vi "Execute Step.vi"(6 "Message Queue":refnum<queue>, 8 "error in (no error)":errorcluster, 9 "Step":T1, 11 "Status":T2) -> (0 "error out":errorcluster, 3 "Status":T2)   [LabVIEW 2012]
doc: "This VI will:\n- confirm that the vehicle is in the correct position\n- update the proper indicators on the console\n- set the vehicle in position light to green\n- indicate the time remaining to the console (continuously update as the step is executing)\n- once the step is complete, the appropriate indicators will be updated (for the steps)\n-- if the vehicle needs to move before more steps can be executed (or at the end of a cycle) exit and set waiting status to vehicle position"
uses:
  Architecture/Message Queue/Message Cluster.ctl
  Architecture/Message Queue/Message Queue.lvlib
  Simulated Console/Controls/Button state.ctl
  Controls/Controller Status.ctl
  Controls/Steps.ctl
  Controls/Stations.ctl
  Controls/Waiting States.ctl
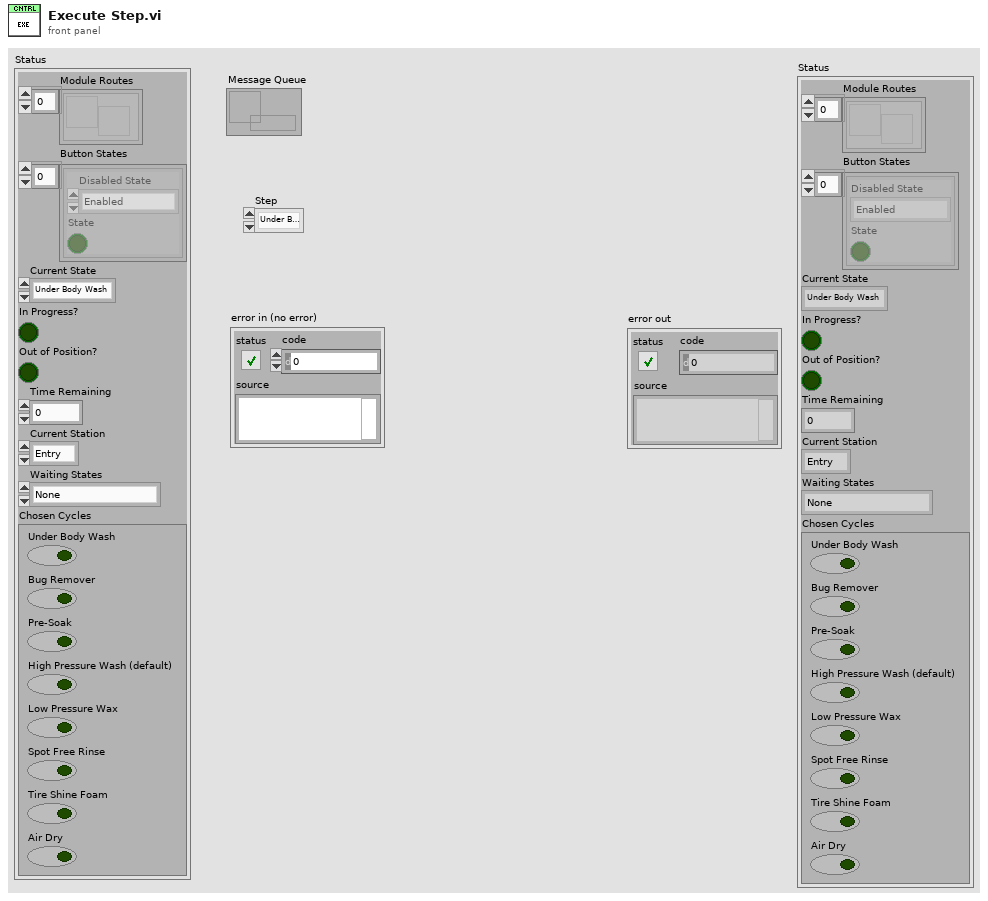
[diagram p1: front panel]
types:
  T1 = typedef "Steps.ctl" = enum16{"Under Body Wash", "Bug Remover", "Pre-Soak", "High Pressure Wash", "Low Pressure Wax", "Spot Free Rinse", "Tire Shine Foam", "Air Dry"}
  T2 = typedef "Controller Status.ctl" = cluster{"Module Routes":refnum<user-event>[], "Button States":T3[], "Current State":T1, "In Progress?":bool, "Out of Position?":bool, "Time Remaining":dbl, "Current Station":T4, "Waiting States":T5, "Chosen Cycles":cluster{"Under Body Wash":bool, "Bug Remover":bool, "Pre-Soak":bool, "High Pressure Wash (default)":bool, "Low Pressure Wax":bool, "Spot Free Rinse":bool, "Tire Shine Foam":bool, "Air Dry":bool}}
  T3 = typedef "Button state.ctl" = cluster{"Disabled State":enum8{"Enabled", "Disabled", "Disabled and Grayed Out"}, "State":bool}
  T4 = typedef "Stations.ctl" = enum16{"Entry", "Station 1", "Station 2", "Station 3", "Exit"}
  T5 = typedef "Waiting States.ctl" = enum16{"None", "for Start", "for Vehicle Position"}
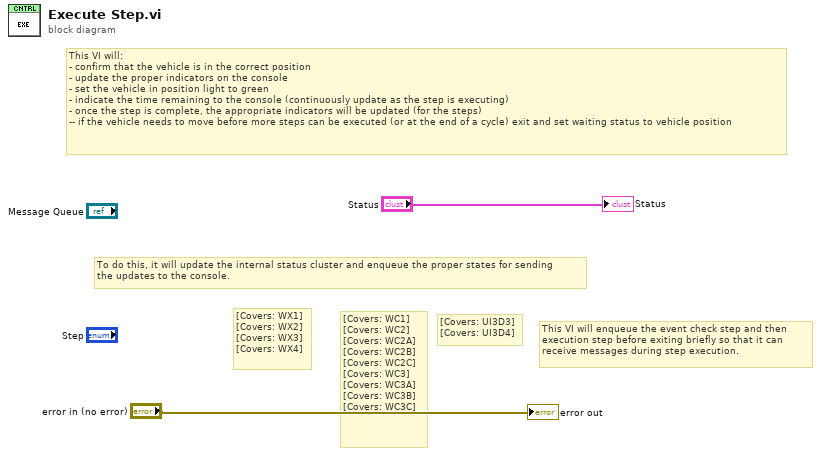
[diagram p0: block diagram]
diagram:
  # "[Covers: UI3D3]\n[Covers: UI3D4]"
  # "This VI will enqueue the event check step and then \nexecution step before exiting briefly so that it can\nreceive messages during step execution."
  # "[Covers: WC1]\n[Covers: WC2]\n[Covers: WC2A]\n[Covers: WC2B]\n[Covers: WC2C]\n[Covers: WC3]\n[Covers: WC3A]\n[Covers: WC3B]\n[Covers: WC3C]"
  # "[Covers: WX1]\n[Covers: WX2]\n[Covers: WX3]\n[Covers: WX4]"
  # "To do this, it will update the internal status cluster and enqueue the proper states for sending\nthe updates to the console."
  # "This VI will:\n- confirm that the vehicle is in the correct position\n- update the proper indicators on the console\n- set the vehicle in position light to green\n- indicate the time remaining to the console (continuously update as the step is executing)\n- once the step is complete, the appropriate indicators will be updated (for the steps)\n-- if the vehicle needs to move before more steps can be executed (or at the end of a cycle) exit and set waiting status to vehicle position"
  "error out" <- "error in (no error)"
  "Status" <- "Status"
